vi "X509_get_common_names.vi"(8 "error in (no error)":errorcluster, 11 "X509-Cert in":refnum<class "X509-Cert.lvclass">) -> (0 "error out":errorcluster, 2 "Cert common names":string[](array[string]), 3 "X509-Cert out":refnum<class "X509-Cert.lvclass">)   [LabVIEW 2013, in "OpenSSL Socket.lvlib" / "X509-Cert.lvclass"]
uses:
  X509-Cert.lvclass
  SSL-Lib/SSL-Lib.lvclass
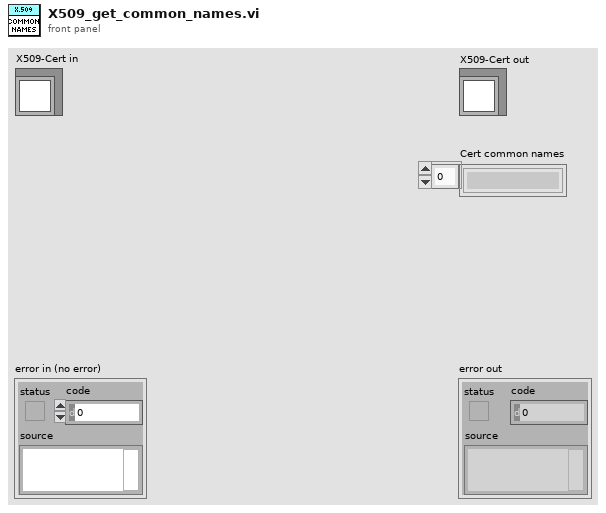
[diagram p1: front panel]
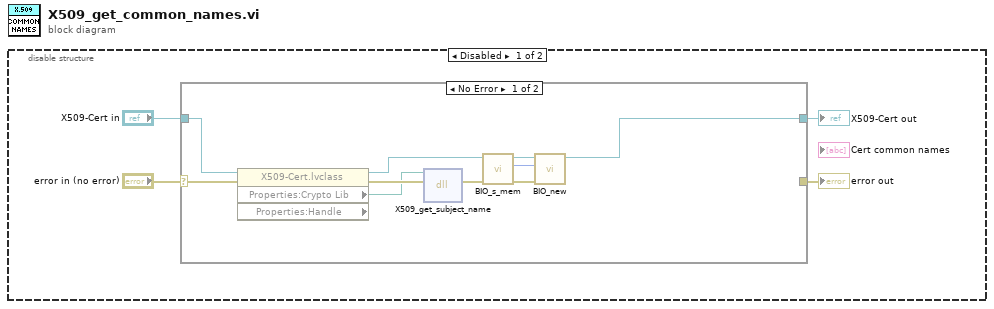
[diagram p0: block diagram]
diagram:
  n1 = disable-structure shown="Disabled" {
    frame Disabled {
      n2 = case shown="No Error" "error in (no error)" {
        selector: "error in (no error)" -> [w15 w18]
        tunnel: [_ w18] -> w3
        tunnel: "X509-Cert in" -> [w16 w17]
        tunnel: [w7 w17] -> w1
        frame No Error {
          n3 = property class="X509-Cert.lvclass" props=["Properties:Crypto Lib", "Properties:Handle"](reference=w16, error in=w15) -> (reference out=w8:refnum<class "X509-Cert.lvclass">, error out=w14:errorcluster, "Properties:Crypto Lib"=w13:path)  [unwired: 1 out]
          n4 = dll-call lib="C:/Program Files (x86)/National Instruments/Shared/nissl/NIlibeay32.dll" fn="X509_get_subject_name"(path in=w13, error in=w14) -> (error out=w9:errorcluster)  [unwired: 4 in, 1 out]
          n5 = call "BIO_s_mem.vi"("error in (no error)"=w9, "SSL-Lib in"=w8) -> ("error out"=w12:errorcluster, "*BIO_Method"=w10:u64, "SSL-Lib out"=w11:refnum<class "X509-Cert.lvclass">)  [unwired: 7 in]
          n6 = call "BIO_new.vi"("error in (no error)"=w12, "*BIO_method"=w10, "SSL-Lib in"=w11) -> ("error out"=w5:errorcluster, "BIO out"=w6:refnum<class "BIO.lvclass">, "SSL-Lib out"=w7:refnum<class "X509-Cert.lvclass">)  [unwired: 6 in]
        }
        frame Error {
        }
      }
      "error out" <- w3
      "X509-Cert out" <- w1
    }
    frame Enabled {
    }
  }
